vi "Actor Core.vi"(8 "error in":errorcluster, 11 "HIJ Vision App IMAQdx Display In":refnum<class "HIJ Vision App IMAQdx Display.lvclass">) -> (0 "error out":errorcluster, 3 "Actor out":refnum<class "Actor.lvclass">)   [LabVIEW 2014, in "HIJ Vision App IMAQdx Display.lvlib" / "HIJ Vision App IMAQdx Display.lvclass"]
doc: "(<B>Filename</B>: Actor Framework.lvlib:Actor.lvclass:Actor Core.vi)\n\nReceives messages to the actor, reacts to them, and initiates any error handling that may shut the actor down.\n\nDescendant classes may override this VI to append parallel tasks for the actor to complete while it handles messages. Overrides use the Call Parent Method node."
uses:
  HIJ Vision App IMAQdx Display.lvclass
  <vilib>/ActorFramework/Actor/Actor.lvclass
  Display Actors/HIJ IMAQdx Display/AF IMAQ Display/HIJ IMAQdx Display.lvclass
  Analyze/Analyze Classes/Analyze Diviation/Analyze BeamDeviation.lvclass
  Analyze/Results and Overlays/Results Beam Deviation/Analyze Results Beam Deviation.lvclass
  Analyze/Analyze Classes/Analyze Distanz/Analyze Distanz.lvclass
  Analyze/Results and Overlays/Results Distance/Analyze Results Distanz.lvclass
  Camera Actors/IMAQdx Actor/IMAQdx Actor/IMAQdx Actor.lvclass
  Display Actors/HIJ Vision Display/HIJ Vision Display/HIJ Vision Display.lvclass/HIJ Vision Display.ctl
  HIJ Vision App IMAQdx Display.lvclass/HIJ Vision App IMAQdx Display.ctl
  HIJ Vision Application/HIJ Vision Application/HIJ Vision Application.lvclass/HIJ Vision Application.ctl
  HIJ Vision Camera App/HIJ Vision Camera App/HIJ Vision Camera App.lvclass/HIJ Vision Camera App.ctl
  Shared Code/Viewable Actor/ViewableActor/ViewableActor.lvclass/ViewableActor.ctl
  <vilib>/ActorFramework/Actor/Actor.lvclass/Actor.ctl
  <vilib>/ActorFramework/Message Enqueuer/Message Enqueuer.lvclass/Message Enqueuer.ctl
  HIJ Vision Camera App/HIJ Vision Camera App Messages/Menu Selection Msg/Menu Selection Msg.lvclass/Menu Selection Msg.ctl
  Display Actors/HIJ Vision Display/HIJ Vision Display/Write Save Report_.vi
  HIJ Vision Application/HIJ Vision Application/Write SubPnl for Display.vi
  HIJ Vision Camera App/HIJ Vision Camera App/Write Child Menu.vi
  HIJ Vision Application/HIJ Vision Application/Write HIJ Vision Display.vi
  HIJ Vision Application/HIJ Vision Application/Write Analyze Objs.vi
  HIJ Vision Camera App/HIJ Vision Camera App/Write Camera Actor.vi
  Shared Code/Viewable Actor/ViewableActor/Write UI VI Ref.vi
  <vilib>/ActorFramework/Message Enqueuer/Init from Existing Queue.vi
  <vilib>/ActorFramework/Message Enqueuer/Enqueue.vi
  <vilib>/ActorFramework/Message Priority Queue/Priority Enqueue.vi
  <vilib>/ActorFramework/Message Enqueuer/Message Enqueuer.lvclass
  HIJ Vision Camera App/HIJ Vision Camera App Messages/Menu Selection Msg/Menu Selection Msg.lvclass
  <vilib>/ActorFramework/Stop Msg/Stop Msg.lvclass
  HIJ Vision Camera App/HIJ Vision Camera App/HIJ Vision Camera App.lvclass
panel:
  in  "Stop Button":bool
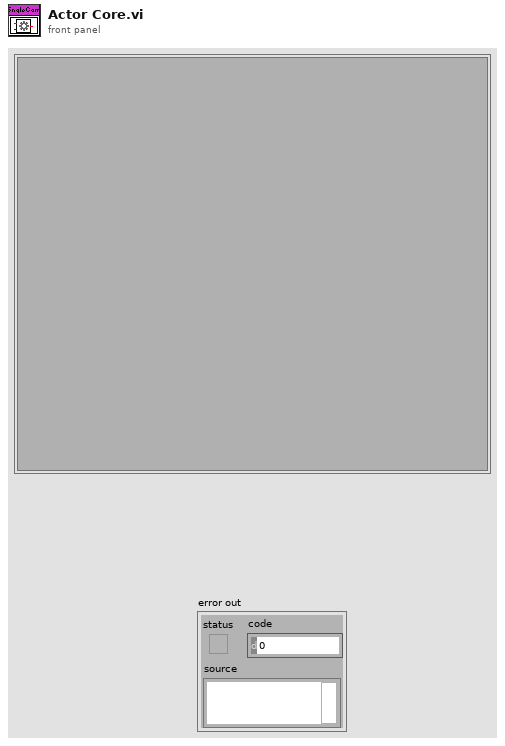
[diagram p1: front panel]
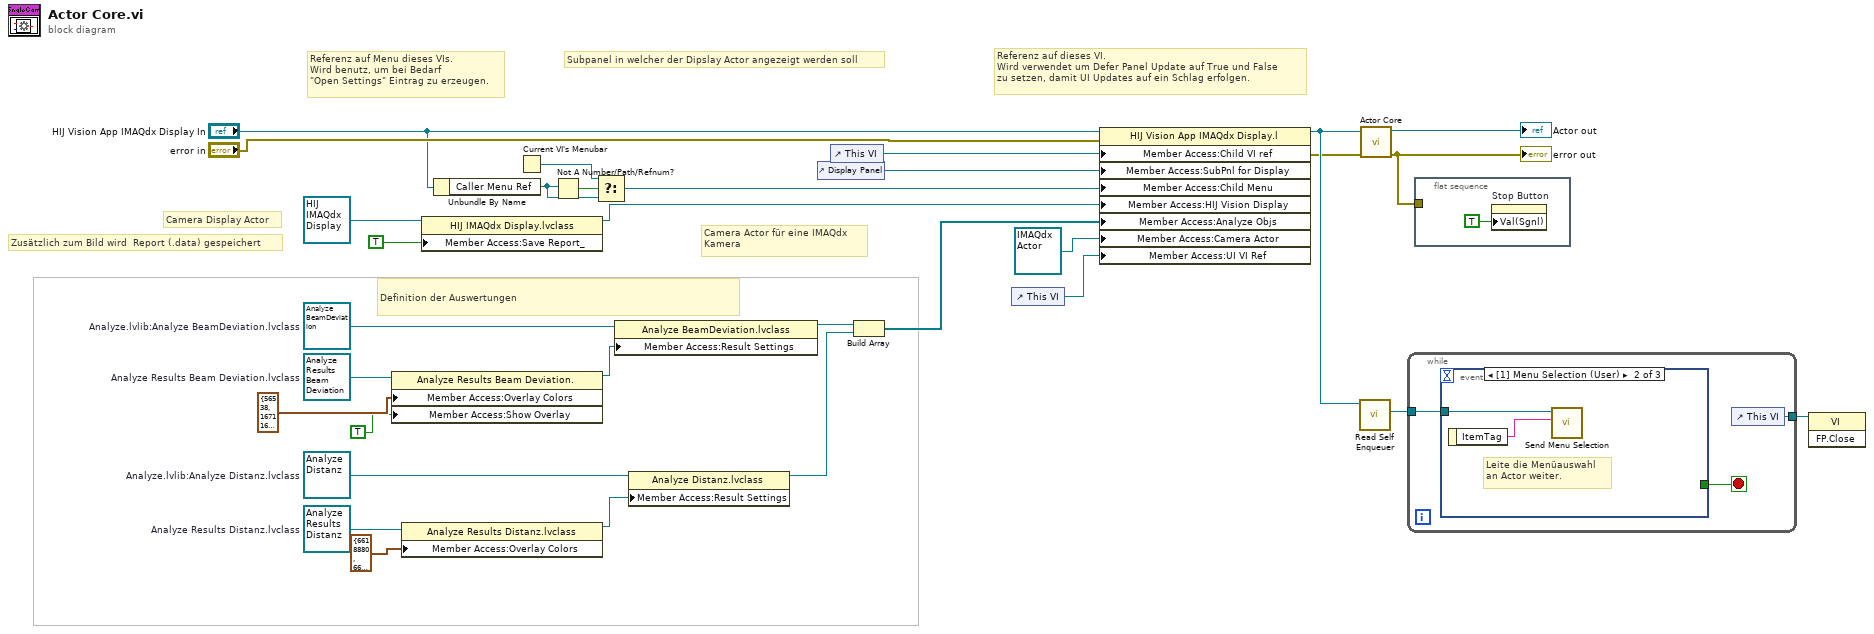
[diagram p0: block diagram]
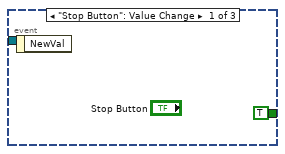
[diagram p2: hidden frame]
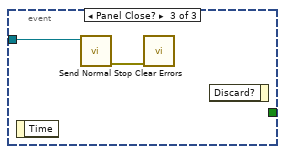
[diagram p3: hidden frame]
diagram:
  w22 = refnum<class "Analyze Results Distanz.lvclass"> refnum  # Analyze Results Distanz.lvclass
  w23 = refnum<class "Analyze Distanz.lvclass"> refnum  # Analyze.lvlib:Analyze Distanz.lvclass
  w25 = refnum<class "Analyze Results Beam Deviation.lvclass"> refnum  # Analyze Results Beam Deviation.lvclass
  w26 = refnum<class "Analyze BeamDeviation.lvclass"> refnum  # Analyze.lvlib:Analyze BeamDeviation.lvclass
  # "Camera Actor für eine IMAQdx\nKamera"
  # "Referenz auf Menu dieses VIs.\nWird benutz, um bei Bedarf \n\"Open Settings\" Eintrag zu erzeugen."
  # "Referenz auf dieses VI.\nWird verwendet um Defer Panel Update auf True und False\nzu setzen, damit UI Updates auf ein Schlag erfolgen."
  # "Definition der Auswertungen"
  # "Camera Display Actor"
  # "Zusätzlich zum Bild wird  Report (.data) gespeichert"
  # "Subpanel in welcher der Dipslay Actor angezeigt werden soll"
  n1 = property class="Analyze Results Beam Deviation."(reference=w25, "Member Access:Overlay Colors"=cluster{"Border":u32, "Text":u32} {"Border"=56538, "Text"=16711680} ("Colors"), "Member Access:Show Overlay"=TRUE ("Show Overlay")) -> (reference out=w11:refnum<class "Analyze Results Beam Deviation.lvclass">)  [unwired: 1 in, 1 out]
  n2 = property class="Analyze Results Distanz.lvclass"(reference=w22, "Member Access:Overlay Colors"=cluster{"Border":u32, "Text":u32} {"Border"=6618880, "Text"=6618880} ("Colors")) -> (reference out=w10:refnum<class "Analyze Results Distanz.lvclass">)  [unwired: 1 in, 1 out]
  n3 = property class="HIJ IMAQdx Display.lvclass"(reference=refnum<class "HIJ IMAQdx Display.lvclass"> refnum ("IMAQ Display.lvlib:IMAQ Display.lvclass"), "Member Access:Save Report_"=TRUE ("Save Report_")) -> (reference out=w13:refnum<class "HIJ IMAQdx Display.lvclass">)  [unwired: 1 in, 1 out]
  n4 = Unbundle By Name("HIJ Vision App IMAQdx Display In") -> ("Caller Menu Ref"=w3:refnum<k9>)
  n5 = Current VI's Menubar() -> (w4:refnum<k9>)
  n6 = Not A Number/Path/Refnum?(number/path/refnum=w3) -> (NaN/Path/Refnum?=w6:bool)
  n7 = Select(t=w4, s=w6, f=w3) -> (s? t:f=w5:refnum<k9>)
  n8 = property class="Analyze BeamDeviation.lvclass"(reference=w26, "Member Access:Result Settings"=w11) -> (reference out=w12:refnum<class "Analyze BeamDeviation.lvclass">)  [unwired: 1 in, 1 out]
  n9 = property class="Analyze Distanz.lvclass"(reference=w23, "Member Access:Result Settings"=w10) -> (reference out=w9:refnum<class "Analyze Distanz.lvclass">)  [unwired: 1 in, 1 out]
  n10 = control-ref of="Display Panel"() -> (w15:refnum<vi>)
  n11 = control-ref of="This VI"() -> (w19:refnum<vi>)
  n12 = Build Array(w12, w9) -> (w16:refnum<class "Analyze BaseClass.lvclass">[])
  n13 = control-ref of="This VI"() -> (w8:refnum<vi>)
  n14 = property class="HIJ Vision App IMAQdx Display.l"(reference="HIJ Vision App IMAQdx Display In", error in="error in", "Member Access:Child VI ref"=w19, "Member Access:SubPnl for Display"=w15, "Member Access:Child Menu"=w5, "Member Access:HIJ Vision Display"=w13, "Member Access:Analyze Objs"=w16, "Member Access:Camera Actor"=refnum<class "IMAQdx Actor.lvclass"> refnum ("IMAQdx Actor.lvlib:IMAQdx Actor.lvclass"), "Member Access:UI VI Ref"=w8) -> (reference out=w20:refnum<class "HIJ Vision App IMAQdx Display.lvclass">, error out=w17:errorcluster)
  n15 = call <vilib>:"Read Self Enqueuer.vi"("Actor"=w20) -> ("Self Enqueuer"=w28:refnum<class "Message Enqueuer.lvclass">)  [unwired: 10 in]
  n16 = call-parent "Actor Core.vi"("error in"=w17, "HIJ Vision Camera App In"=w20) -> ("error out"=w29:errorcluster, "Actor out"=→"Actor out":refnum<class "Actor.lvclass">)  [unwired: 8 in]
  "error out" <- w29
  n17 = while {
    tunnel: w28 -> [w33]
    tunnel: [w32] -> w1
    stop <- w34 stop-if-true
    n18 = event shown="[1] Menu Selection (User)" {
      selector: _ -> [_ _ _]
      dyn-events: _ -> [_ _ _]
      timeout: _ -> [_ _ _]
      tunnel: [TRUE _ _] -> w34
      tunnel: w33 -> [_ w36 w39]
      event "Stop Button": Value Change {
        n19 = event-data() -> ()  [unwired: 1 in, 1 out]
      }
      event Menu Selection (User) {
        # "Leite die Menüauswahl \nan Actor weiter."
        n20 = event-data() -> ("ItemTag"=w37:string)  [unwired: 1 in]
        n21 = call "Send Menu Selection.vi"("MenuTag"=w37, "Message Enqueuer"=w36) -> ()  [unwired: 8 in, 2 out]
      }
      event Panel Close? {
        n22 = event-data() -> ()  [unwired: 1 in, 1 out]
        n23 = call <vilib>:"Send Normal Stop.vi"("Message Enqueuer"=w39) -> ("error out"=w38:errorcluster)  [unwired: 10 in]
        n24 = call <vilib>:"Clear Errors.vi"("error in (no error)"=w38) -> ()  [unwired: 5 in, 2 out]
        n25 = event-data() -> ()  [unwired: 2 in, 1 out]
      }
    }
    n26 = control-ref of="This VI"() -> (w32:refnum<vi>)
  }
  n27 = flat-sequence {
    tunnel: w29 -> [_]
    frame #0 {
      n28 = property on="Stop Button" class="Bool (strict)"("Val(Sgnl)"=TRUE) -> ()  [unwired: 2 in, 2 out]
    }
  }
  n29 = invoke class="VI" method="FP.Close"(reference=w1) -> ()  [unwired: 2 in, 3 out]
